vi "Actor Core.vi"(8 "error in":errorcluster, 11 "Sample PWM Fans in":refnum<class "Sample PWM Fans.lvclass">) -> (0 "error out":errorcluster, 3 "Actor out":refnum<class "Actor.lvclass">)   [LabVIEW 2023, in "Sample PWM Fans.lvlib" / "Sample PWM Fans.lvclass"]
doc: "(<B>Filename</B>: Actor Framework.lvlib:Actor.lvclass:Actor Core.vi)\n\nReceives messages to the actor, reacts to them, and initiates any error handling that may shut the actor down.\n\nDescendant classes may override this VI to append parallel tasks for the actor to complete while it handles messages. Overrides use the Call Parent Class Method node."
uses:
  Sample PWM Fans.lvclass
  <vilib>/ActorFramework/Actor/Actor.lvclass
  Sample PWM Fans.lvclass/Sample PWM Fans.ctl
  <vilib>/ActorFramework/Message Enqueuer/Message Enqueuer.lvclass/Message Enqueuer.ctl
  Series/ISeries Actor/ISeries Actor Messages/Do Task Msg/Do Task Msg.lvclass/Do Task Msg.ctl
  <vilib>/ActorFramework/Message Enqueuer/Enqueue.vi
  Series/ISeries Actor/ISeries Actor Messages/Stop Tasks Msg/Stop Tasks Msg.lvclass
  Series/ISeries Actor/ISeries Actor Messages/Start Tasks Msg/Start Tasks Msg.lvclass
  <vilib>/ActorFramework/Stop Msg/Stop Msg.lvclass
  Series/ISeries Actor/ISeries Actor Messages/Do Task Msg/Do Task Msg.lvclass
  <vilib>/Utility/LVClass/Get LV Class Name.vi
  <resource>/AFDebug/Generate Trace for Message.vi
  <vilib>/ActorFramework/Message Priority Queue/Priority Enqueue.vi
  Series/Series Actor/Series Actor/Series Actor.lvclass
  <vilib>/MGI/Panel Manager/Panel Actor/Panel Actor/Panel Actor.lvclass
panel:
  out "Remote Setpoint F1":dbl format="%#_g %"
  out "Remote Setpoint F2":dbl format="%#_g %"
  in  "Kill Series Button":bool
  in  "Start Button":bool
  in  "Stop Button":bool
  in  "Fan2":dbl(knob) scale=0.0..100.0 scale format="%#_g %"
  in  "Fan1":dbl(knob) scale=0.0..100.0 scale format="%#_g %"
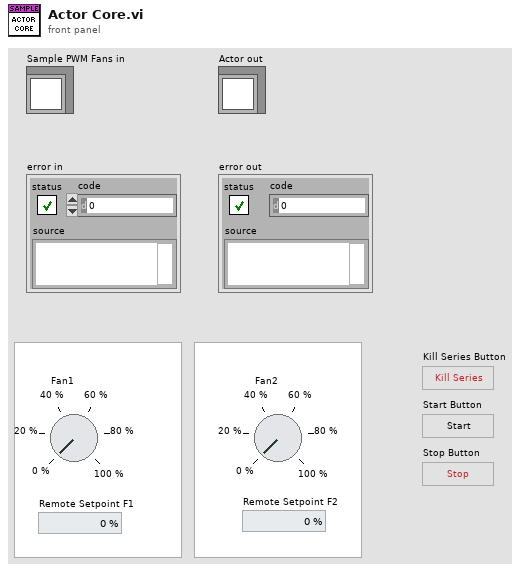
[diagram p1: front panel]
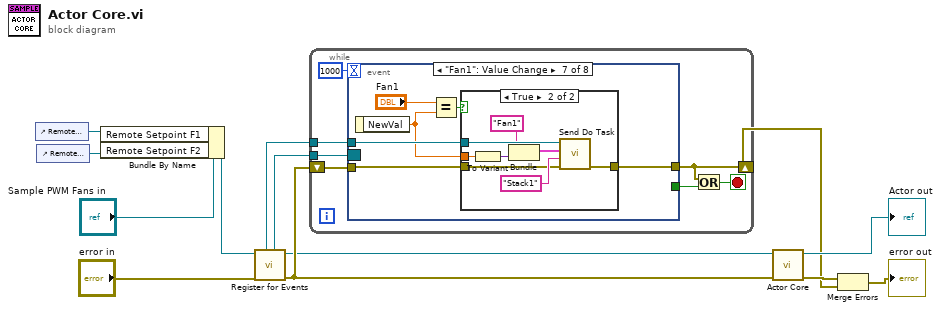
[diagram p0: block diagram]
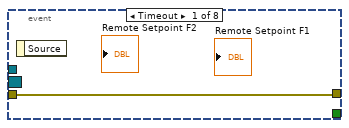
[diagram p2: hidden frame]
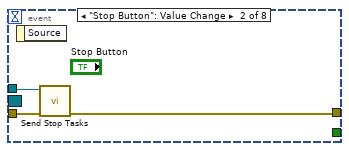
[diagram p3: hidden frame]
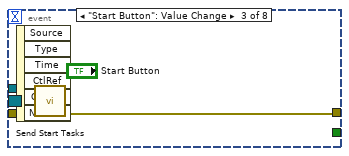
[diagram p4: hidden frame]
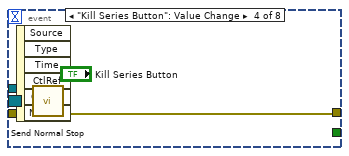
[diagram p5: hidden frame]
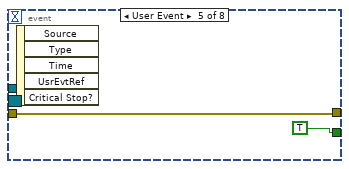
[diagram p6: hidden frame]
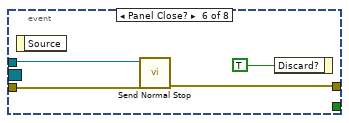
[diagram p7: hidden frame]
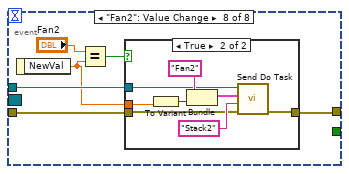
[diagram p9: hidden frame]
diagram:
  n1 = control-ref of="Remote Setpoint F1"() -> (w7:refnum<vi>)
  n2 = control-ref of="Remote Setpoint F2"() -> (w8:refnum<vi>)
  n3 = Bundle By Name(cluster="Sample PWM Fans in", "Remote Setpoint F1"=w7, "Remote Setpoint F2"=w8) -> (w5:refnum<class "Sample PWM Fans.lvclass">)
  n4 = call <vilib>:"Register for Events.vi"("Error In"="error in", "Panel Actor in"=w5) -> ("Error Out"=w4:errorcluster, "Panel Actor out"=w3:refnum<class "Sample PWM Fans.lvclass">, "Pnl Actor"=w1:refnum<event-registration>, "Self Enqueuer"=w2:refnum<class "Message Enqueuer.lvclass">)  [unwired: 6 in]
  n5 = while {
    tunnel: w2 -> [w20]
    shift-right: [w15] -> w9
    shift-left: w4 -> [w19]
    tunnel: w1 -> [w14]
    stop <- w16 stop-if-true
    n6 = event shown="[6] \"Fan1\": Value Change" {
      selector: w14 -> [_ _ _ _ _ _ _ _]
      dyn-events: _ -> [_ _ _ _ _ _ _ _]
      timeout: 1000 -> [_ _ _ _ _ _ _ _]
      tunnel: w20 -> [_ w23 w26 w29 _ w34 w39 w56]
      tunnel: w19 -> [w21 w24 w27 w30 w31 w35 w40 w55]
      tunnel: [_ _ _ _ TRUE _ _ _] -> w18
      tunnel: [w21 w22 w25 w28 w31 w33 w37 w52] -> w15
      event Timeout {
        n7 = event-data() -> ()  [unwired: 1 in, 1 out]
      }
      event "Stop Button": Value Change {
        n8 = event-data() -> ()  [unwired: 1 in, 1 out]
        n9 = call "Send Stop Tasks.vi"("error in (no error)"=w24, "Message Enqueuer"=w23) -> ("error out"=w22:errorcluster)  [unwired: 8 in, 1 out]
      }
      event "Start Button": Value Change {
        n10 = event-data() -> ()  [unwired: 1 in, 6 out]
        n11 = call "Send Start Tasks.vi"("error in (no error)"=w27, "Message Enqueuer"=w26) -> ("error out"=w25:errorcluster)  [unwired: 8 in, 1 out]
      }
      event "Kill Series Button": Value Change {
        n12 = event-data() -> ()  [unwired: 1 in, 6 out]
        n13 = call <vilib>:"Send Normal Stop.vi"("error in (no error)"=w30, "Message Enqueuer"=w29) -> ("error out"=w28:errorcluster)  [unwired: 9 in]
      }
      event User Event {
        n14 = event-data() -> ()  [unwired: 1 in, 5 out]
      }
      event Panel Close? {
        n15 = event-data() -> ()  [unwired: 1 in, 1 out]
        n16 = call <vilib>:"Send Normal Stop.vi"("error in (no error)"=w35, "Message Enqueuer"=w34) -> ("error out"=w33:errorcluster)  [unwired: 9 in]
        n17 = event-data("Discard?"=TRUE) -> ()  [unwired: 1 in, 1 out]
      }
      event "Fan1": Value Change {
        n18 = event-data() -> ("NewVal"=w38:dbl)  [unwired: 1 in]
        n19 = Equal?(x="Fan1", y=w38) -> (x = y?=w41:bool)
        n20 = case shown="True" w41 {
          tunnel: w39 -> [_ w49]
          tunnel: w40 -> [w43 w48]
          tunnel: w38 -> [_ w44]
          tunnel: [w43 w51] -> w37
          frame False {
          }
          frame True {
            n21 = To Variant(anything=w44) -> (Variant=w45:variant)
            n22 = Bundle("Fan1", "Variant"=w45) -> (w47:cluster{string, "Variant":variant})  [unwired: 1 in]
            n23 = call "Send Do Task.vi"("error in (no error)"=w48, "Task Ident"="Stack1", "Input"=w47, "Message Enqueuer"=w49) -> ("error out"=w51:errorcluster)  [unwired: 6 in, 1 out]
          }
        }
      }
      event "Fan2": Value Change {
        n24 = event-data() -> ("NewVal"=w53:dbl)  [unwired: 1 in]
        n25 = Equal?(x="Fan2", y=w53) -> (x = y?=w54:bool)
        n26 = case shown="True" w54 {
          tunnel: w56 -> [_ w60]
          tunnel: w55 -> [w58 w61]
          tunnel: w53 -> [_ w59]
          tunnel: [w58 w62] -> w52
          frame False {
          }
          frame True {
            n27 = To Variant(anything=w59) -> (Variant=w63:variant)
            n28 = Bundle("Fan2", "Variant"=w63) -> (w65:cluster{string, "Variant":variant})  [unwired: 1 in]
            n29 = call "Send Do Task.vi"("error in (no error)"=w61, "Task Ident"="Stack2", "Input"=w65, "Message Enqueuer"=w60) -> ("error out"=w62:errorcluster)  [unwired: 6 in, 1 out]
          }
        }
      }
    }
    n30 = Or(x=w15, y=w18) -> (x .or. y?=w16:bool)
  }
  n31 = call-parent "Actor Core.vi"("error in"=w4, "Series Actor in"=w3) -> ("error out"=w13:errorcluster, "Actor out"=→"Actor out":refnum<class "Actor.lvclass">)  [unwired: 8 in]
  n32 = Merge Errors(w13, w9) -> (→"error out":errorcluster)
